vi "Init Data.vi"(8 "error in (no error)":errorcluster, 11 "VacuumLine in":refnum<class "VacuumLine.lvclass">) -> (0 "error out":errorcluster, 3 "VacuumLine out":refnum<class "VacuumLine.lvclass">)   [LabVIEW 2016, in "Hardware.lvlib" / "VacuumLine.lvlib" / "VacuumLine.lvclass"]
uses:
  <userlib>/Common Components/Hardware/Abstract System/VacuumLine/VacuumLine/VacuumLine.lvclass
  <userlib>/Common Components/Hardware/Abstract System/VacuumLine/VacuumLine/Error States.ctl
  <userlib>/Common Components/Hardware/Abstract System/VacuumLine/VacuumLine/VacuumLine.lvclass/VacuumLine.ctl
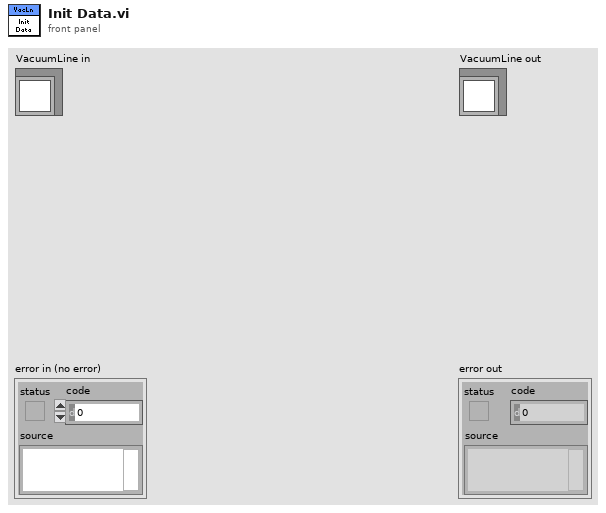
[diagram p1: front panel]
types:
  T1 = typedef "Hardware.lvlib/VacuumLine.lvlib/VacuumLine.lvclass/Error States.ctl" = cluster{"Pos out of range?":bool, "Motor Pos & DispSnsr asynced?":bool, "Hitting Valve?":bool[], "Sample Car left in Valve (decoupled)?":bool[], "Optical Switch malfunction":bool[], "Motor disconnected":bool, "DispSnsr disconnected":bool, "LogicIO disconnected":bool}
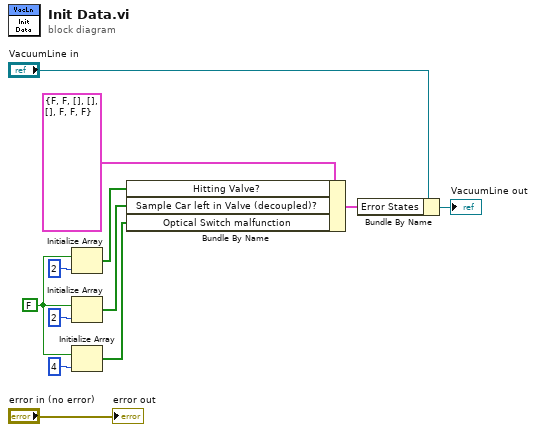
[diagram p0: block diagram]
diagram:
  w2 = FALSE
  n1 = Initialize Array(w2, 2 ("dimension size")) -> (w6:bool[])
  n2 = Initialize Array(w2, 2 ("dimension size")) -> (w4:bool[])
  n3 = Initialize Array(w2, 4 ("dimension size")) -> (w1:bool[])
  n4 = Bundle By Name(cluster=T1 {"Pos out of range?"=FALSE, "Motor Pos & DispSnsr asynced?"=FALSE, "Hitting Valve?"=[], "Sample Car left in Valve (decoupled)?"=[], "Optical Switch malfunction"=[], "Motor disconnected"=FALSE, "DispSnsr disconnected"=FALSE, "LogicIO disconnected"=FALSE} ("Error States"), "Hitting Valve?"=w6, "Sample Car left in Valve (decoupled)?"=w4, "Optical Switch malfunction"=w1) -> (w8:T1)
  n5 = Bundle By Name(cluster="VacuumLine in", "Error States"=w8) -> (→"VacuumLine out":refnum<class "VacuumLine.lvclass">)
  "error out" <- "error in (no error)"
